vi "Rohde & Schwarz VNA Fetch Data.vi"(6 "Channel":i8=1 min=1 max=99 step=1, 7 "Rohde & Schwarz VNA":T2, 8 "error in (no error)":errorcluster, 9 "Formatted Data?":bool, 10 "Data to Read (Data)":enum16{"Data", "Memory"}(ring), 11 "VISA Resource Name":refnum<visa-resource-name>) -> (0 "error out":errorcluster, 1 "Display Format":T1, 2 "Data (real+imag)":cdb[](array[numeric]), 3 "dup VISA Resource Name":refnum<visa-resource-name>)   [LabVIEW 2011]
doc: "It is recommended that you hold off triggers before running this VI as the HP8753 tends to \"hang\" if data is read while measurements are being taken.\n\n This VI is used to collect and display data generated by the HP8753 Network Analyzer. The VI can display error-corrected data, error-corrected trace memory, fully formatted data and memory traces. For further information on these types of data see Processsing Chain figure in the HPIB programming note. When the data type is a formatted data, the instruments screen will change to reflect what is being displayed, eg. selecting \"formatted memory\" changes the display to \"MEMORY\".\n\n The data values shown depend upon the data type and the measurement format. If the data type is \"error-corrected data\" or \"error-corrected trace memory\" and/or the measurement format is \"Smith chart\" or \"polar\", the data values are real,imaginary pairs. Otherwise the data values are stimulus,response pairs. These pairs correspond to what is shown in the graphical display.\n\n Data can also be saved to a file with this VI. When saving a file, the stimulus is always shown. The real,imaginary components or the response value are also shown depending upon the data type and the measurement format. \n\n No units are shown on the VI front panel or in the data file. All units are basic units of Hz, dB, seconds, ohms, etc. The \"saved data comments\" control should be used for any special information such as the measurement format, averaging and smoothing information, etc.\n\n Whether or not data is saved and whether the output is in real,imaginary pairs or stimulus,response parirs affects the speed of this VI. When data is saved to a file and/or when data is in stimulus,response pairs, requires the reading of the stimulus values which slows the VI down. The fastest reads are done when the data type is \"error-corrected data\" or \"error-corrected trace memory\" and/or the measurement format is \"Smith chart\" or \"polar\" and data is not being saved to a file.\n\n This VI sets the format, ie. linear or logarithmic, depending upon the sweep type. \n\nFYI - Originally this VI was written without considering the stimulus values. In most case this would be fine for display purposes as the point number could be used for the X value as most sweeps are evenly spaced. This is not the case with frequency list sweeps which can have big gaps in the sweep. For this reason the stimulus value is read (at least in the cases explained above) to make the LabVIEW display match what is display on the instrument's display."
uses:
  TypeDefs/Rohde & Schwarz VNA Instrument Info.ctl
  tests/S Parameter/TypeDefs/SP Measurement Format.ctl
panel:
  out "Waveform Graph":dbl[](graph)
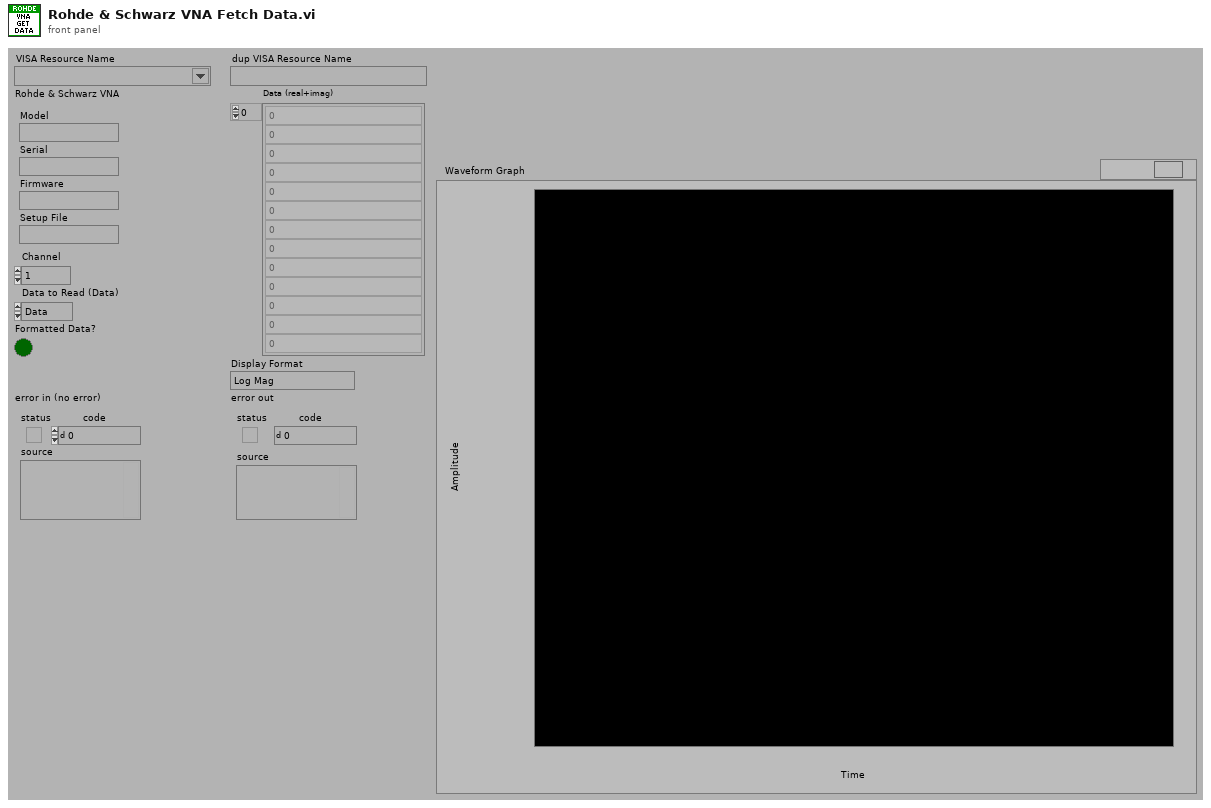
[diagram p1: front panel]
types:
  T1 = typedef "SP Measurement Format.ctl" = enum32{"Log Mag", "Phase", "Delay", "Smith (R+jX)", "Polar (Re/Im)", "Linear Mag", "SWR", "Real", "Imaginary", "Smith (Lin/Phase)", "Smith (Log/Phase)", "Smith (Real/Imag)", "Smith (G+jB)", "Polar (Lin/Phase)", "Polar (Log/Phase)", "Expanded Phase", "Positive Phase", "Inverted Smith", "Unwrapped Phase", "Power Out", "Power In", "Linear Mag/Phase", "Log Mag/Phase", "Real/Imaginary"}
  T2 = typedef "Rohde & Schwarz VNA Instrument Info.ctl" = cluster{"Model":string, "Serial":string, "Firmware":string, "Setup File":string}
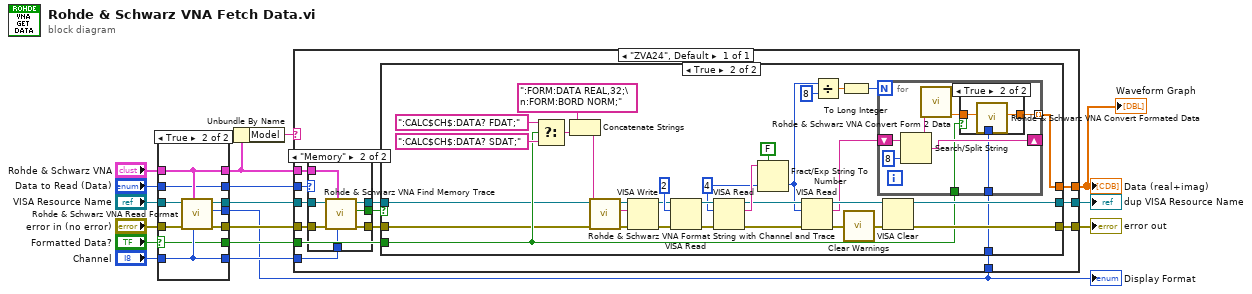
[diagram p0: block diagram]
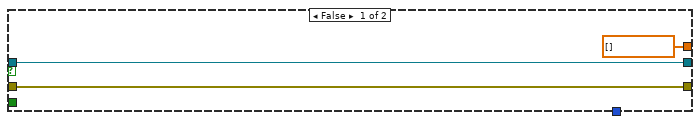
[diagram p3: hidden frame]
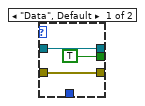
[diagram p5: hidden frame]
diagram:
  n1 = case shown="True" "Formatted Data?" {
    selector: "Formatted Data?" -> [w18 w24]
    tunnel: "error in (no error)" -> [w23 w32]
    tunnel: "VISA Resource Name" -> [w22 w31]
    tunnel: [w22 w30] -> w13
    tunnel: [w23 w29] -> w12
    tunnel: "Rohde & Schwarz VNA" -> [w21 w28]
    tunnel: "Channel" -> [w20 w27]
    tunnel: [w21 w28] -> w3
    tunnel: [w20 w27] -> w9
    tunnel: "Data to Read (Data)" -> [w19 w26]
    tunnel: [w19 w26] -> w7
    tunnel: [_ w25] -> w2
    tunnel: [w18 w24] -> w5
    frame False {
    }
    frame True {
      n2 = call "Rohde & Schwarz VNA Read Format.vi"("Channel"=w27, "Rohde & Schwarz VNA"=w28, "error in (no error)"=w32, "VISA Resource Name"=w31) -> ("error out"=w29:errorcluster, "Display Format"=w25:T1, "dup VISA Resource Name"=w30:refnum<visa-resource-name>)  [unwired: 5 out]
    }
  }
  "Display Format" <- w2
  n3 = Unbundle By Name(w3) -> ("Model"=w4:string)
  n4 = case shown="\"ZVA24\", Default" w4 {
    tunnel: w13 -> [w41]
    tunnel: w12 -> [w40]
    tunnel: [w44] -> w17
    tunnel: [w43] -> w1
    tunnel: [w45] -> w16
    tunnel: w7 -> [w35]
    tunnel: w9 -> [w36]
    tunnel: w5 -> [w42]
    tunnel: w3 -> [w37]
    tunnel: w2 -> [w33]
    frame "ZVA24", Default {
      n5 = case shown="\"Memory\"" w35 {
        tunnel: w41 -> [w93 w101]
        tunnel: w40 -> [w94 w100]
        tunnel: [w94 w99] -> w39
        tunnel: [w93 w98] -> w38
        tunnel: w37 -> [_ w97]
        tunnel: w36 -> [_ w96]
        tunnel: [TRUE ("Memory Exists?") w95] -> w34
        frame "Data", Default {
        }
        frame "Memory" {
          n6 = call "Rohde & Schwarz VNA Find Memory Trace.vi"("Channel"=w96, "Rohde & Schwarz VNA"=w97, "error in (no error)"=w100, "VISA Resource Name"=w101) -> ("error out"=w99:errorcluster, "Memory Exists?"=w95:bool, "dup VISA Resource Name"=w98:refnum<visa-resource-name>)  [unwired: 5 out]
        }
      }
      n7 = case shown="True" w34 {
        tunnel: [w47 w68] -> w45
        tunnel: [w48 w67] -> w44
        tunnel: [cdb[] [] w61] -> w43
        tunnel: w33 -> [_ w60]
        tunnel: w42 -> [_ w57]
        tunnel: w39 -> [w48 w52]
        tunnel: w38 -> [w47 w51]
        frame False {
        }
        frame True {
          w72 = u32 4
          n8 = Select(t=":CALC$CH$:DATA? FDAT;" ("String"), s=w57, f=":CALC$CH$:DATA? SDAT;" ("String")) -> (s? t:f=w55:string)
          n9 = Concatenate Strings(":FORM:DATA REAL,32;\n:FORM:BORD NORM;" ("String"), w55) -> (w54:string)
          n10 = call "Rohde & Schwarz VNA Format String with Channel and Trace.vi"("String"=w54) -> ("String Out"=w53:string)  [unwired: 2 in, 6 out]
          n11 = VISA Write(VISA resource name=w51, write buffer=w53, error in (no error)=w52) -> (VISA resource name out=w78:refnum<visa-resource-name>, error out=w77:errorcluster)  [unwired: 1 out]
          n12 = VISA Read(VISA resource name=w78, byte count=u32 2, error in (no error)=w77) -> (VISA resource name out=w76:refnum<visa-resource-name>, error out=w75:errorcluster)  [unwired: 2 out]
          n13 = VISA Read(VISA resource name=w76, byte count=w72, error in (no error)=w75) -> (VISA resource name out=w66:refnum<visa-resource-name>, read buffer=w73:string, error out=w65:errorcluster)  [unwired: 1 out]
          n14 = Fract/Exp String To Number(use system decimal point (T)=FALSE, string=w73, default (0 dbl)=w72) -> (number=w64:u32)  [unwired: 2 out]
          n15 = VISA Read(VISA resource name=w66, byte count=w64, error in (no error)=w65) -> (VISA resource name out=w63:refnum<visa-resource-name>, read buffer=w62:string, error out=w50:errorcluster)  [unwired: 1 out]
          n16 = Divide(x=w64, y=u32 8) -> (x/y=w70:dbl)
          n17 = To Long Integer(number=w70) -> (32bit integer=w69:i32)
          n18 = call "Clear Warnings.vi"("error in (no error)"=w50) -> ("error out"=w49:errorcluster)
          n19 = for {
            N: w69 -> [_]
            shift-right: [w84] -> _
            shift-left: w62 -> [w85]
            tunnel: [w82] -> w61 mode=indexing
            tunnel: w60 -> [w81]
            tunnel: w57 -> [w80]
            n20 = Search/Split String(string=w85, offset (0)=8) -> (substring before match=w83:string, match + rest of string=w84:string)  [unwired: 2 out]
            n21 = call "Rohde & Schwarz VNA Convert Form 2 Data.vi"("Raw Data Point"=w83) -> ("Number"=w87:cdb)  [unwired: 10 out]
            n22 = case shown="True" w80 {
              tunnel: w87 -> [w88 w90]
              tunnel: [w88 w89] -> w82
              tunnel: w81 -> [_ w91]
              frame False {
              }
              frame True {
                n23 = call "Rohde & Schwarz VNA Convert Formated Data.vi"("Display Format"=w91, "Number"=w90) -> ("Number"=w89:cdb)  [unwired: 9 out]
              }
            }
          }
          n24 = VISA Clear(VISA resource name=w63, error in (no error)=w49) -> (VISA resource name out=w68:refnum<visa-resource-name>, error out=w67:errorcluster)
        }
      }
    }
  }
  "dup VISA Resource Name" <- w16
  "error out" <- w17
  "Data (real+imag)" <- w1
  "Waveform Graph" <- w1
